vi "Write Sub Panel Message.vi"(8 "error in (no error)":errorcluster, 10 "Sub Panel Message":refnum<vi>, 11 "MSG in":refnum<class "MSG.lvclass">) -> (0 "error out":errorcluster, 3 "MSG out":refnum<class "MSG.lvclass">)   [LabVIEW 2020, in "MSG.lvlib" / "MSG.lvclass"]
uses:
  MSG.lvclass
  MSG.lvclass/MSG.ctl
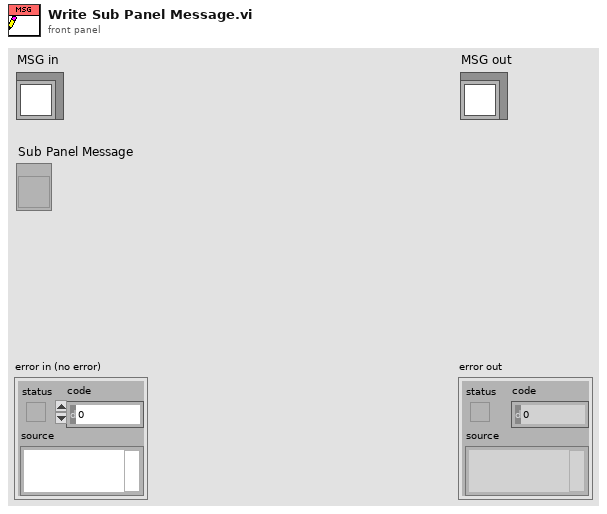
[diagram p1: front panel]
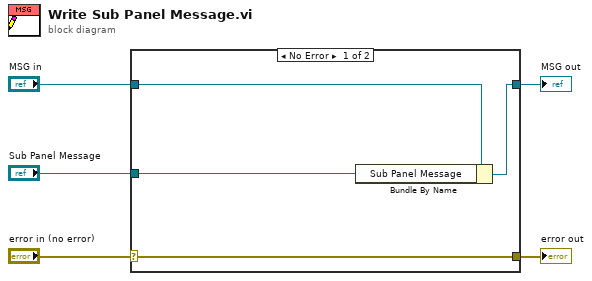
[diagram p0: block diagram]
diagram:
  n1 = case shown="No Error" "error in (no error)" {
    selector: "error in (no error)" -> [w9 w10]
    tunnel: [w9 w10] -> w4
    tunnel: [w7 w11] -> w2
    tunnel: "MSG in" -> [w8 w11]
    tunnel: "Sub Panel Message" -> [w6 _]
    frame No Error {
      n2 = Bundle By Name(cluster=w8, "Sub Panel Message"=w6) -> (w7:refnum<class "MSG.lvclass">)
    }
    frame Error {
    }
  }
  "error out" <- w4
  "MSG out" <- w2
